vi "Expand and Index Button States.vi"(2 "Button Index":i32, 3 "Button States":refnum<class "Button.lvclass">[](array[class])) -> (0 "Button.lvclass":refnum<class "Button.lvclass">, 1 "Button States Out":refnum<class "Button.lvclass">[](array[class]))   [LabVIEW 2012, in "Toolbar.xctl"]
doc: "Essentailly the same as indexing the array of button isntances, but ensures that the button instance array is big enough to include the requested index (i.e. creating extra buttons at the end of the array if needed)."
uses:
  Toolbar.xctl
  Button_Class/Button.lvclass
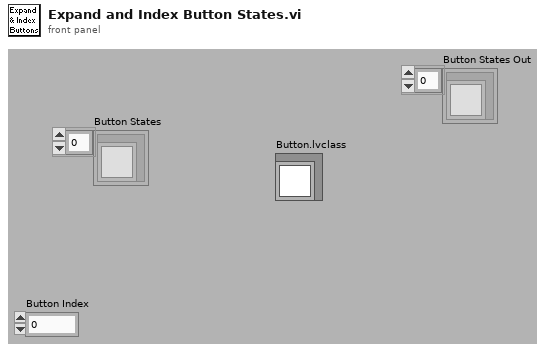
[diagram p1: front panel]
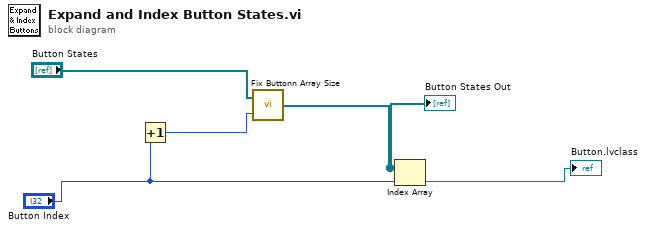
[diagram p0: block diagram]
diagram:
  n1 = Increment(x="Button Index") -> (x+1=w1:i32)
  n2 = call "Fix Buttonn Array Size.vi"("Number of Buttons"=w1, "Button States In"="Button States") -> ("Button States Out"=w2:refnum<class "Button.lvclass">[])
  "Button States Out" <- w2
  n3 = Index Array(array=w2, index="Button Index") -> (element=→"Button.lvclass":refnum<class "Button.lvclass">)
